vi "LSTRLotNoRxToLot.vi"(8 "Boolean":bool=TRUE, 10 "String":string) -> (2 "before match":string)   [LabVIEW 2012]
uses:
  <vilib>/regexp/Match Regular Expression.xnode
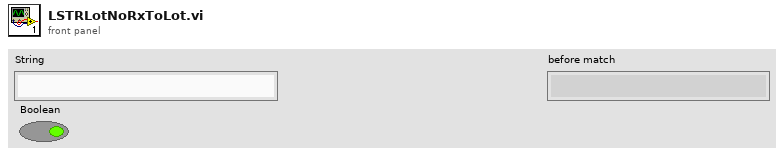
[diagram p1: front panel]
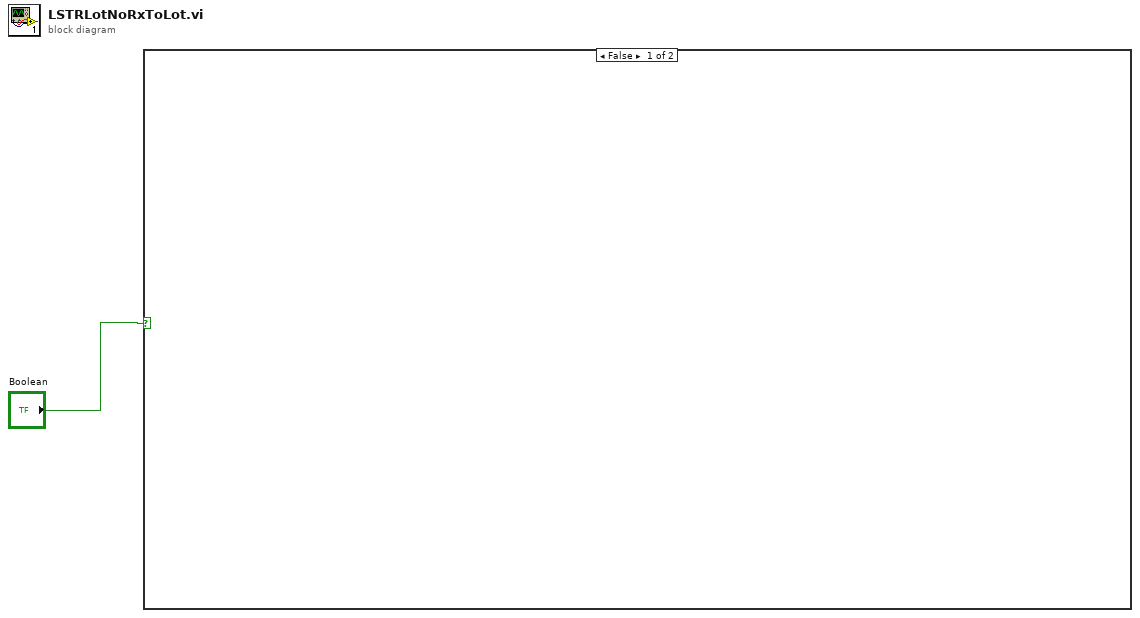
[diagram p0: block diagram]
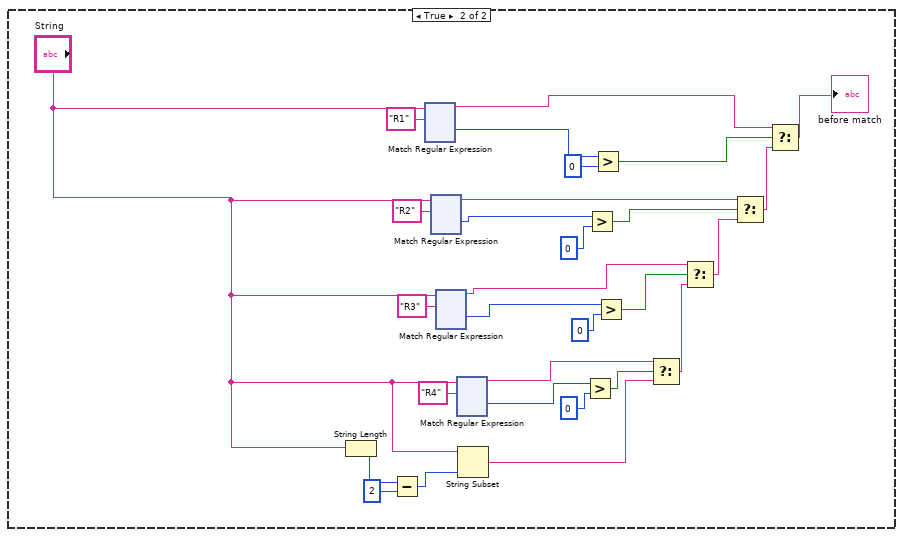
[diagram p2: hidden frame]
diagram:
  n1 = case shown="False" "Boolean" {
    frame False {
    }
    frame True {
      n2 = String Length(string="String") -> (length=w5:i32)
      n3 = Subtract(x=w5, y=2) -> (x-y=w3:i32)
      n4 = xnode "Match Regular Expression"("input string"="String", "regular expression"="R1") -> ("before match"=w17:string, "offset past match"=w26:i32)  [unwired: 4 in, 3 out]
      n5 = xnode "Match Regular Expression"("input string"="String", "regular expression"="R2") -> ("before match"=w13:string, "offset past match"=w19:i32)  [unwired: 4 in, 3 out]
      n6 = xnode "Match Regular Expression"("input string"="String", "regular expression"="R3") -> ("before match"=w10:string, "offset past match"=w20:i32)  [unwired: 4 in, 3 out]
      n7 = xnode "Match Regular Expression"("input string"="String", "regular expression"="R4") -> ("before match"=w8:string, "offset past match"=w21:i32)  [unwired: 4 in, 3 out]
      n8 = String Subset(string="String", length (rest)=w3) -> (substring=w2:string)  [unwired: 1 in]
      n9 = Greater?(x=w21, y=0) -> (0:w7:bool)
      n10 = Greater?(x=w19, y=0) -> (0:w14:bool)
      n11 = Greater?(x=w26, y=0) -> (0:w18:bool)
      n12 = Greater?(x=w20, y=0) -> (0:w11:bool)
      n13 = Select(t=w8, s=w7, f=w2) -> (s? t:f=w9:string)
      n14 = Select(t=w10, s=w11, f=w9) -> (s? t:f=w12:string)
      n15 = Select(t=w13, s=w14, f=w12) -> (s? t:f=w15:string)
      n16 = Select(t=w17, s=w18, f=w15) -> (s? t:f=→"before match":string)
    }
  }
